vi "RF_step.vi"(4 "RF Range 2":cluster{"Numeric":i32, "Numeric 2":i32}, 6 "RF Range 1":cluster{"Numeric":i32, "Numeric 2":i32}, 8 "RF Step Value":i32, 9 "2 ranges?":bool, 10 "RF on":bool, 11 "RF Location":i32) -> (2 "RF Indicator":bool, 3 "RF Location out":i32)   [LabVIEW 2018]
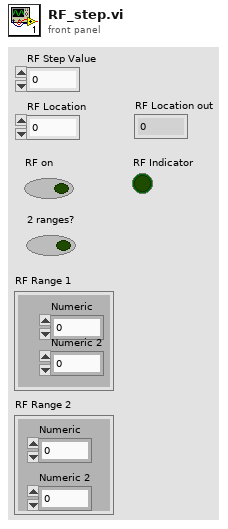
[diagram p1: front panel]
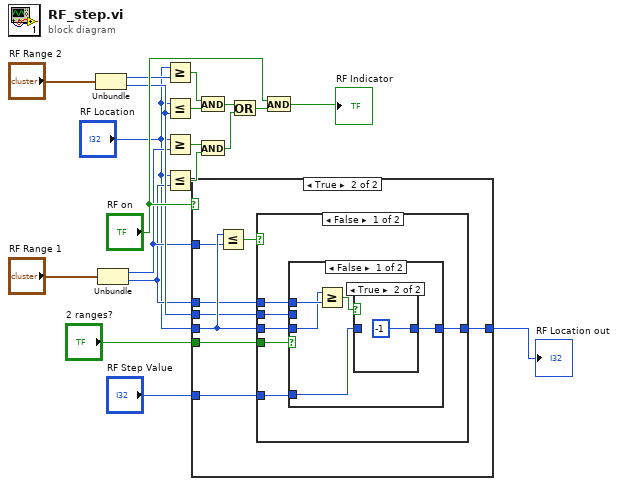
[diagram p0: block diagram]
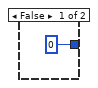
[diagram p2: hidden frame]
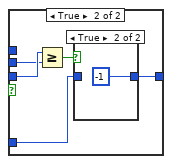
[diagram p4: hidden frame]
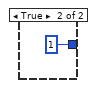
[diagram p6: hidden frame]
diagram:
  n1 = Unbundle("RF Range 2") -> ("Numeric"=w7:i32, "Numeric 2"=w6:i32)
  n2 = Unbundle("RF Range 1") -> ("Numeric"=w5:i32, "Numeric 2"=w4:i32)
  n3 = Greater Or Equal?(x="RF Location", y=w7) -> (x >= y?=w11:bool)
  n4 = Less Or Equal?(x="RF Location", y=w6) -> (x <= y?=w8:bool)
  n5 = Greater Or Equal?(x="RF Location", y=w5) -> (x >= y?=w10:bool)
  n6 = Less Or Equal?(x="RF Location", y=w4) -> (x <= y?=w9:bool)
  n7 = case shown="True" "RF on" {
    tunnel: "2 ranges?" -> [_ w28]
    tunnel: "RF Location" -> [_ w25]
    tunnel: [0 w26] -> w18
    tunnel: w5 -> [_ w24]
    tunnel: w4 -> [_ w23]
    tunnel: w6 -> [_ w22]
    tunnel: "RF Step Value" -> [_ w21]
    frame False {
    }
    frame True {
      n8 = Less Or Equal?(x=w25, y=w24) -> (x <= y?=w27:bool)
      n9 = case shown="False" w27 {
        tunnel: w28 -> [w34 _]
        tunnel: [w31 1] -> w26
        tunnel: w23 -> [w33 _]
        tunnel: w25 -> [w32 _]
        tunnel: w22 -> [w30 _]
        tunnel: w21 -> [w29 _]
        frame False {
          n10 = case shown="False" w34 {
            tunnel: w33 -> [w39 _]
            tunnel: w32 -> [w36 w44]
            tunnel: [w37 w45] -> w31
            tunnel: w30 -> [_ w43]
            tunnel: w29 -> [w35 w42]
            frame False {
              n11 = Greater Or Equal?(x=w36, y=w39) -> (x >= y?=w38:bool)
              n12 = case shown="True" w38 {
                tunnel: [w40 -1] -> w37
                tunnel: w35 -> [w40 _]
                frame False {
                }
                frame True {
                }
              }
            }
            frame True {
              n13 = Greater Or Equal?(x=w44, y=w43) -> (x >= y?=w46:bool)
              n14 = case shown="True" w46 {
                tunnel: [w47 -1] -> w45
                tunnel: w42 -> [w47 _]
                frame False {
                }
                frame True {
                }
              }
            }
          }
        }
        frame True {
        }
      }
    }
  }
  "RF Location out" <- w18
  n15 = And(x=w11, y=w8) -> (x .and. y?=w13:bool)
  n16 = And(x=w10, y=w9) -> (x .and. y?=w12:bool)
  n17 = Or(x=w13, y=w12) -> (x .or. y?=w15:bool)
  n18 = And(x="RF on", y=w15) -> (x .and. y?=→"RF Indicator":bool)
